vi "Launch ExampleDependency.vi"(8 "error in (no error)":errorcluster, 9 "Name":string="ExampleDependency", 11 "SMO.Example in":refnum<class "SMO.Example.lvclass">) -> (0 "error out":errorcluster, 1 "Dependency Name":string, 2 "Dependency Reference":refnum<class "SMO.lvclass">, 3 "SMO.Example out":refnum<class "SMO.Example.lvclass">)   [LabVIEW 2013, in "SMO.Example.lvclass"]
uses:
  SMO.Example.lvclass
  src/SMO/SMO.lvclass
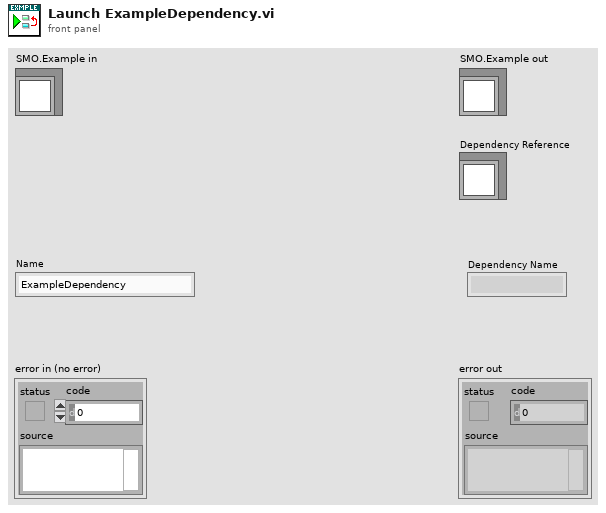
[diagram p1: front panel]
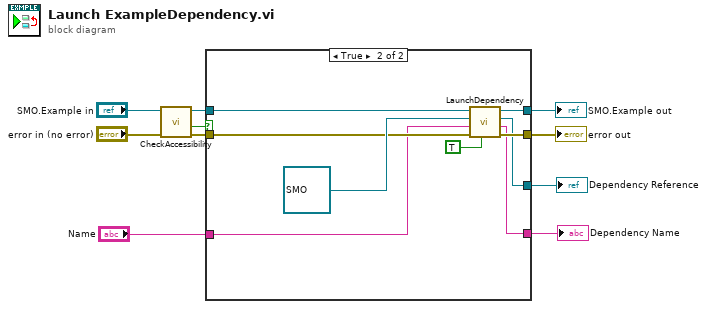
[diagram p0: block diagram]
diagram:
  n1 = call "CheckAccessibility.vi"("error in (no error)"="error in (no error)", "SMO in"="SMO.Example in") -> ("error out"=w7:errorcluster, "Accessible"=w4:bool, "SMO out"=w5:refnum<class "SMO.Example.lvclass">)  [unwired: 7 in]
  n2 = case shown="True" w4 {
    tunnel: [w11 w21] -> w10
    tunnel: [w12 w20] -> w9
    tunnel: w7 -> [w11 w17]
    tunnel: w5 -> [w12 w16]
    tunnel: [_ w15] -> w3
    tunnel: "Name" -> [_ w14]
    tunnel: [_ w13] -> w1
    frame False {
    }
    frame True {
      n3 = call "LaunchDependency.vi"("Shared Resource"=TRUE, "error in (no error)"=w17, "Dependency Name"=w14, "Dependency Type"=refnum<class "SMO.lvclass"> refnum ("SMO.lvclass"), "SMO in"=w16) -> ("error out"=w21:errorcluster, "Unique Name"=w13:string, "Dependency Reference"=w15:refnum<class "SMO.lvclass">, "SMO out"=w20:refnum<class "SMO.Example.lvclass">)  [unwired: 3 in]
    }
  }
  "error out" <- w10
  "SMO.Example out" <- w9
  "Dependency Reference" <- w3
  "Dependency Name" <- w1
